vi "user32_MoveWindow.vi"(4 "nHeight":i32, 5 "y":i32, 6 "nWidth":i32, 7 "x":i32, 8 "error in (no error)":errorcluster, 10 "BRePaint":i32, 11 "hWnd":i64) -> (0 "error out":errorcluster, 3 "Return Value":i32)   [LabVIEW 2020]
uses:
  user32.dll
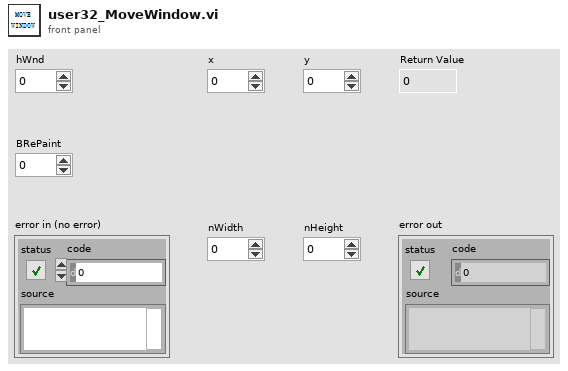
[diagram p1: front panel]
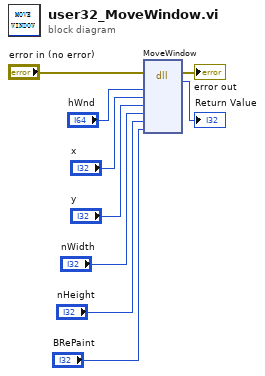
[diagram p0: block diagram]
diagram:
  n1 = dll-call lib="user32.dll" fn="MoveWindow"(error in="error in (no error)", "hWnd"="hWnd", "x"="x", "y"="y", "nWidth"="nWidth", "nHeight"="nHeight", "BRePaint"="BRePaint") -> (error out=→"error out":errorcluster, "返回值"=→"Return Value":i32)  [unwired: 8 in, 1 out]
